vi "LSMcontroller_v64_updatedwaveformhandling.vi"() -> ()   [LabVIEW 2015] (continued)
                                tunnel: [_ w2837 _ w2843] -> w2785
                                frame 1 {
                                n478 = call "2pparameters.vi"("command"="get") -> ("params out"=w2797:T10)  [unwired: 1 in]
                                n479 = Unbundle By Name(w2797) -> ("wavdet"=w2798:bool, "sAOxy"=w2800:i32, "refwfsize"=w2801:dbl, "srate Img"=w2799:sgl)
                                n480 = call "waveformsDObuffer.vi"("command"="get") -> ("DO wf out"=w2793:digitalwaveform[])  [unwired: 1 in]
                                n481 = case shown="True" w2798 {
                                tunnel: [w2805 w2818] -> w2795
                                tunnel: w2799 -> [w2814 w2833]
                                tunnel: w2800 -> [w2804 w2824]
                                tunnel: w2801 -> [_ w2830]
                                frame False {
                                w2808 = u16 0 items=["unsigned binary", "offset binary", "2's complement"] ("data format (offset binary)")
                                n482 = Initialize Array(sgl 0.0, w2804) -> (w2811:sgl[])
                                n483 = Replace Array Subset(array=w2811, new element=sgl 1.0, index=0) -> (w2809:sgl[])
                                n484 = Reciprocal(x=w2814) -> (1/x=w2815:sgl)
                                n485 = Bundle By Name("Y"=w2809, "dt"=w2815) -> (w2806:waveform(sgl))  [unwired: 1 in]
                                n486 = call-poly <vilib>:"Analog to Digital.vi"("data format (offset binary)"=w2808, "compress digital (T)"=TRUE, "full-scale range (pk-pk)"=1.0, "resolution (16 bit)"=1, "analog waveform"=w2806) -> ("digital waveform"=w2805:digitalwaveform)  [unwired: 3 in, 3 out]
                                }
                                frame True {
                                w2821 = u16 0 items=["unsigned binary", "offset binary", "2's complement"] ("data format (offset binary)")
                                n487 = To Double Precision Float(number=w2824) -> (double precision float=w2831:dbl)
                                n488 = Initialize Array(sgl 0.0, w2824) -> (w2826:sgl[])
                                n489 = Divide(x=w2830, y=w2831) -> (x/y=w2828:dbl)
                                n490 = Round Toward +Infinity(x=w2828) -> (ceil(x): smallest int >= x=w2829:dbl)
                                n491 = Replace Array Subset(array=w2826, new element=sgl 1.0, index=0) -> (w2823:sgl[])
                                n492 = for {
                                N: w2829 -> [_]
                                tunnel: w2823 -> [w2835]
                                tunnel: [w2835] -> w2832 mode=concatenating
                                }
                                n493 = Reciprocal(x=w2833) -> (1/x=w2834:sgl)
                                n494 = Bundle By Name("Y"=w2832, "dt"=w2834) -> (w2819:waveform(sgl))  [unwired: 1 in]
                                n495 = call-poly <vilib>:"Analog to Digital.vi"("data format (offset binary)"=w2821, "compress digital (T)"=TRUE, "full-scale range (pk-pk)"=1.0, "resolution (16 bit)"=1, "analog waveform"=w2819) -> ("digital waveform"=w2818:digitalwaveform)  [unwired: 3 in, 3 out]
                                }
                                }
                                n496 = Build Array (concatenate)(w2793, w2795) -> (w2791:digitalwaveform[])
                                n497 = call "waveformsDObuffer.vi"("DO wf in"=w2791, "command"="set") -> ()  [unwired: 1 out]
                                }
                                frame 2 {
                                n498 = call "waveformsDObuffer.vi"("command"="get") -> ("DO wf out"=w2839:digitalwaveform[])  [unwired: 1 in]
                                n499 = Delete From Array(array=w2839, length=1, index=w2842) -> (deleted portion=w2837:digitalwaveform[], array with subset deleted=w2836:digitalwaveform[])
                                n500 = call "waveformsDObuffer.vi"("DO wf in"=w2836, "command"="set") -> ()  [unwired: 1 out]
                                }
                                frame 3, Default {
                                }
                                frame 0 {
                                n501 = local read "Measurement"() -> (w2845:T4)
                                n502 = To Unsigned Long Integer(number=w2845) -> (unsigned 32bit integer=w2844:u32)
                                n503 = case shown="5..7" w2844 {
                                tunnel: w2846 -> [_ w2849]
                                tunnel: [_ w2848] -> w2843
                                frame 0..4, Default {
                                }
                                frame 5..7 {
                                n504 = call "2pparameters.vi"("command"="get") -> ("params out"=w2856:T10)  [unwired: 1 in]
                                n505 = Unbundle By Name(w2856) -> ("wavdet"=w2857:bool, "sAOxy"=w2859:i32, "refwfsize"=w2860:dbl, "srate Img"=w2858:sgl)
                                n506 = call "waveformsDObuffer.vi"("command"="get") -> ("DO wf out"=w2850:digitalwaveform[])  [unwired: 1 in]
                                n507 = Index Array(array=w2850, index=w2849) -> (element=w2851:digitalwaveform)
                                n508 = case shown="True" w2857 {
                                tunnel: [w2864 w2877] -> w2854
                                tunnel: w2858 -> [w2873 w2892]
                                tunnel: w2859 -> [w2863 w2883]
                                tunnel: w2860 -> [_ w2889]
                                frame False {
                                w2867 = u16 0 items=["unsigned binary", "offset binary", "2's complement"] ("data format (offset binary)")
                                n509 = Initialize Array(sgl 0.0, w2863) -> (w2870:sgl[])
                                n510 = Replace Array Subset(array=w2870, new element=sgl 1.0, index=0) -> (w2868:sgl[])
                                n511 = Reciprocal(x=w2873) -> (1/x=w2874:sgl)
                                n512 = Bundle By Name("Y"=w2868, "dt"=w2874) -> (w2865:waveform(sgl))  [unwired: 1 in]
                                n513 = call-poly <vilib>:"Analog to Digital.vi"("data format (offset binary)"=w2867, "compress digital (T)"=TRUE, "full-scale range (pk-pk)"=1.0, "resolution (16 bit)"=1, "analog waveform"=w2865) -> ("digital waveform"=w2864:digitalwaveform)  [unwired: 3 in, 3 out]
                                }
                                frame True {
                                w2880 = u16 0 items=["unsigned binary", "offset binary", "2's complement"] ("data format (offset binary)")
                                n514 = To Double Precision Float(number=w2883) -> (double precision float=w2890:dbl)
                                n515 = Initialize Array(sgl 0.0, w2883) -> (w2885:sgl[])
                                n516 = Divide(x=w2889, y=w2890) -> (x/y=w2887:dbl)
                                n517 = Round Toward +Infinity(x=w2887) -> (ceil(x): smallest int >= x=w2888:dbl)
                                n518 = Replace Array Subset(array=w2885, new element=sgl 1.0, index=0) -> (w2882:sgl[])
                                n519 = for {
                                N: w2888 -> [_]
                                tunnel: w2882 -> [w2894]
                                tunnel: [w2894] -> w2891 mode=concatenating
                                }
                                n520 = Reciprocal(x=w2892) -> (1/x=w2893:sgl)
                                n521 = Bundle By Name("Y"=w2891, "dt"=w2893) -> (w2878:waveform(sgl))  [unwired: 1 in]
                                n522 = call-poly <vilib>:"Analog to Digital.vi"("data format (offset binary)"=w2880, "compress digital (T)"=TRUE, "full-scale range (pk-pk)"=1.0, "resolution (16 bit)"=1, "analog waveform"=w2878) -> ("digital waveform"=w2877:digitalwaveform)  [unwired: 3 in, 3 out]
                                }
                                }
                                n523 = Build Array(w2851) -> (w2848:digitalwaveform[])
                                n524 = Replace Array Subset(array=w2850, new element=w2854, index=w2849) -> (w2847:digitalwaveform[])
                                n525 = call "waveformsDObuffer.vi"("DO wf in"=w2847, "command"="set") -> ()  [unwired: 1 out]
                                }
                                }
                                }
                                }
                              }
                              frame #10 {
                                n526 = local read "Meastab"() -> (w2909:enum32{"X-Y Image", "Linescan", "Timetrace"})
                                n527 = property on="refwf" class="Ring (strict)"() -> ("RingText.Text"=w2906:string)  [unwired: 2 in, 2 out]
                                n528 = case shown="\"Timetrace\"" w2909 {
                                tunnel: [w2911 w2912] -> w2910
                                frame "X-Y Image", Default {
                                n529 = local read "Sampling rate"() -> (w2911:dbl)
                                }
                                frame "Timetrace" {
                                n530 = local read "srateAODOtt"() -> (w2912:dbl)
                                }
                                }
                                n531 = call "waveformsAObuffer.vi"("command"="get") -> ("AO wf out"=w2897:waveform(dbl)[])  [unwired: 1 in]
                                n532 = local read "wavdet"() -> (w2907:bool)
                                n533 = call "waveformsDObuffer.vi"("command"="get") -> ("DO wf out"=w2901:digitalwaveform[])  [unwired: 1 in]
                                n534 = call "correctwaveformsizetemp.vi"("new sampling frequency (Hz)"=w2910, "start"=TRUE, "reference waveforms to"=w2906, "Analog waveforms in"=w2897, "stop"=FALSE, "Digital waveforms in"=w2901) -> ("analog wf out"=w2903:waveform(dbl)[], "Digital wf out"=w2905:digitalwaveform[], "measpoints"=w2908:i32)
                                n535 = call "GetNumCamFramesv2.vi"("Digital Waveform Graph"=w2905) -> ("Numeric"=w2904:i32)  [unwired: 10 in]
                                n536 = call "waveformsDObuffer.vi"("DO wf in"=w2905, "command"="set") -> ()  [unwired: 1 out]
                                n537 = call "waveformsAObuffer.vi"("AO wf in"=w2903, "command"="set") -> ()  [unwired: 1 out]
                                n538 = local write "Total Camera Frames"(w2904) -> ()
                                n539 = case shown="True" w2907 {
                                tunnel: w2908 -> [_ w2913]
                                frame False {
                                }
                                frame True {
                                n540 = local write "# of frames"(w2913) -> ()
                                }
                                }
                              }
                            }
                          }
                          frame #6 {
                            # "Disabled for conversion to 64 bit"
                            n541 = disable-structure shown="Disabled" {
                              frame Disabled {
                                n542 = local read "Measurement"() -> (w2918:T4)
                                n543 = case shown="\"Lifetime (scan)\"" w2918 {
                                frame "X-Y-t movie", Default {
                                }
                                frame "Lifetime (scan)" {
                                # "total acquisition time"
                                n544 = call "2pparameters.vi"("command"="get") -> ("params out"=w2924:T10)  [unwired: 1 in]
                                n545 = Unbundle By Name(w2924) -> ("measpoints"=w2945:i32, "avpp"=w2946:i32, "sAOxy"=w2925:i32, "srate Img"=w2947:sgl)
                                n546 = Multiply(x=w2945, y=w2946) -> (x*y=w2943:i32)
                                n547 = To Double Precision Float(number=w2925) -> (double precision float=w2930:dbl)
                                n548 = Divide(x=w2930, y=w2947) -> (x/y=w2932:dbl)
                                n549 = To Double Precision Float(number=w2943) -> (double precision float=w2928:dbl)
                                n550 = local read "min phot"() -> (w2939:u32)
                                n551 = local read "expected c/s"() -> (w2940:dbl)
                                n552 = Multiply(x=w2928, y=w2932) -> (x*y=w2926:dbl)
                                n553 = Multiply(x=w2926, y=1000.0) -> (x*y=w2931:dbl)
                                n554 = local read "Ch1 ZeroX"() -> (w2937:i32)
                                n555 = local read "truncate"() -> (w2938:u32)
                                n556 = To Long Integer(number=w2931) -> (32bit integer=w2941:i32)
                                n557 = To Long Integer(number=w2940) -> (32bit integer=w2942:i32)
                                n558 = local read "Number of Bins"() -> (w2933:u32)
                                n559 = local read "Ch1 Level"() -> (w2935:i32)
                                n560 = local read "Ch0 ZeroX"() -> (w2936:i32)
                                n561 = local write "Acquisition time"(w2941) -> ()
                                n562 = local read "Ch0 Level"() -> (w2934:i32)
                                n563 = call "lifetimeparameters.vi"("command"="get") -> ("Params out"=w2922:T19)  [unwired: 1 in]
                                n564 = Add(x=10, y=w2941) -> (x+y=w2929:i32)
                                n565 = Bundle By Name(cluster=w2922, "acq time"=w2929, "acq rate"=w2942, "# bins"=w2933, "Ch0 Level"=w2934, "Ch1 Level"=w2935, "Ch0 ZeroX"=w2936, "Ch1 ZeroX"=w2937, "min photons"=w2939, "truncate"=w2938) -> (w2921:T19)
                                n566 = local write "Acquisition rate"(w2942) -> ()
                                n567 = call "lifetimeparameters.vi"("Params in"=w2921, "command"="set") -> ()  [unwired: 1 out]
                                }
                                }
                                n568 = local read "min phot"() -> (w2916:u32)
                                n569 = Decrement(x=w2916) -> (x-1=w2917:u32)
                                n570 = To Double Precision Float(number=w2917) -> (double precision float=w2915:dbl)
                                n571 = property on="img_CH1" class="IntGraph (strict)"("ZScale.Minimum"=w2915) -> ()  [unwired: 2 in, 2 out]
                              }
                              frame Enabled {
                              }
                            }
                            n572 = local write "64bit disabled"(TRUE ("64bit disabled")) -> ()
                          }
                          frame #7 {
                            n573 = local read "Sampling rate"() -> (w2949:dbl)
                            n574 = call "calcdaqtime.vi"("sampling rate"=w2949) -> ("Calc. time per frame (ms)"=w2948:dbl)
                            n575 = local write "Calc. time per frame (ms)"(w2948) -> ()
                          }
                          frame #8 {
                            n576 = call "2pparameters.vi"("command"="get") -> ("params out"=w2960:T10)  [unwired: 1 in]
                            n577 = local read "Measurement"() -> (w2951:T4)
                            n578 = Unbundle By Name(w2960) -> ("bufferAI"=w2958:i32, "srate"=w2959:sgl)
                            n579 = To Double Precision Float(number=w2958) -> (double precision float=w2952:dbl)
                            n580 = To Double Precision Float(number=w2959) -> (double precision float=w2962:dbl)
                            n581 = case shown="\"X-Y-t movie\", Default" w2951 {
                              tunnel: [w2967 w2971] -> w2950
                              frame "X-Y-t movie", Default {
                                n582 = local read "wavdet"() -> (w2968:bool)
                                n583 = case shown="False" w2968 {
                                tunnel: [w2969 w2970] -> w2967
                                frame False {
                                w2969 = 10123 items=["Finite Samples"=10178, "Continuous Samples"=10123, "Hardware Timed Single Point"=12522] ("sample mode")
                                }
                                frame True {
                                w2970 = 10123 items=["Finite Samples"=10178, "Continuous Samples"=10123, "Hardware Timed Single Point"=12522] ("sample mode")
                                }
                                }
                              }
                              frame "X-Y-Z stack" {
                                w2971 = 10178 items=["Finite Samples"=10178, "Continuous Samples"=10123, "Hardware Timed Single Point"=12522] ("sample mode")
                              }
                            }
                            n584 = Divide(x=w2952, y=w2962) -> (x/y=w2966:dbl)
                            n585 = Multiply(x=w2966, y=2.0) -> (x*y=w2963:dbl)
                            n586 = Max & Min(x=w2963, y=10.0) -> (max(x,y)=w2953:dbl)  [unwired: 1 out]
                            n587 = call "2pparameters.vi"("command"="get") -> ("params out"=w2957:T10)  [unwired: 1 in]
                            n588 = Bundle By Name(cluster=w2957, "timeout"=w2953, "sample mode"=w2950) -> (w2954:T10)
                            n589 = call "2pparameters.vi"("Params in"=w2954, "command"="set") -> ()  [unwired: 1 out]
                          }
                          frame #9 {
                            n590 = local read "# of frames"() -> (w2972:i32)
                            n591 = call "timestamps.vi"("# of frames"=w2972, "command"="init") -> ()  [unwired: 2 in, 1 out]
                          }
                        }
                      }
                      frame #2 {
                        # "Disabled for conversion to 64 bit"
                        n592 = call "prepAO_img.vi"() -> ("Terminal Name with Device Prefix"=w2975:tag)
                        n593 = call "prepAI_img.vi"("triggersource"=w2975) -> ()  [unwired: 2 in]
                        n594 = call "prepCI_img.vi"("ArmStart.DigEdge.Src"=w2975) -> ()  [unwired: 1 in]
                        n595 = call "prepDO_img.vi"() -> ()  [unwired: 2 in]
                        n596 = disable-structure shown="Disabled" {
                          frame Disabled {
                            n597 = local read "Measurement"() -> (w2976:T4)
                            n598 = case shown="\"Lifetime (scan)\"" w2976 {
                              frame "X-Y-t movie", Default {
                              }
                              frame "Lifetime (scan)" {
                                n599 = stacked-sequence {
                                frame #0 {
                                n600 = call "PH-temp.vi"("String"="clear" ("command")) -> ()  [unwired: 2 in, 2 out]
                                n601 = call "PH-temp-raw.vi"("command"="empty") -> ()  [unwired: 1 in, 1 out]
                                }
                                frame #1 {
                                n602 = call "calib.vi"() -> ()  [unwired: 1 in]
                                }
                                frame #2 {
                                n603 = call "setup.vi"() -> ()  [unwired: 1 in]
                                }
                                }
                              }
                            }
                          }
                          frame Enabled {
                          }
                        }
                        n604 = local write "64bit disabled"(TRUE ("64bit disabled")) -> ()
                      }
                      frame #3 {
                        n605 = local read "save\ndata"() -> (w2979:bool)
                        n606 = case shown="True" w2979 {
                          tunnel: w2980 -> [_ w2984]
                          frame False {
                          }
                          frame True {
                            n607 = local read "filename prefix"() -> (w2982:string)
                            n608 = local read "data dir"() -> (w2983:path)
                            n609 = call "preparetiffs.vi"("filename prefix"=w2982, "data dir"=w2983, "timestamp"=w2984) -> ("full-filename"=w2981:string)  [unwired: 1 in]
                            n610 = local write "full-filename"(w2981) -> ()
                          }
                        }
                        n611 = call "preptempbuffers.vi"() -> ()  [unwired: 12 in]
                      }
                      frame #4 {
                        # "Disabled Thorlabs Zstage;\nneeds to be replaced by PI code"
                        n612 = local read "Measurement"() -> (w2985:T4)
                        n613 = case shown="\"X-Y-Z stack\"" w2985 {
                          frame "X-Y-t movie", Default {
                          }
                          frame "X-Y-Z stack" {
                            # "Move Z stage"
                            n614 = stacked-sequence {
                              seq-local: [w2987 _] -> [_ w3000]
                              frame #0 {
                                n615 = local read "Z-Start (um)"() -> (w2991:dbl)
                                n616 = local read "Z-end (um)"() -> (w2990:dbl)
                                n617 = local read "# of frames"() -> (w2992:i32)
                                n618 = call "calcZslice.vi"("current slice"=0, "# of Slices"=w2992, "Z-Start (um)"=w2991, "Z-end (um)"=w2990) -> ("zpos (V)"=w2988:dbl, "zpos (um)"=w2987:dbl)
                                n619 = call "moveZ_V2.vi"("Z"=w2988) -> ()
                                n620 = local write "Cal. Z"(w2987) -> ()
                              }
                              frame #1 {
                                n621 = local read "Pstart"() -> (w2999:dbl)
                                n622 = local read "Pend"() -> (w2998:dbl)
                                n623 = local read "exp?"() -> (w2997:bool)
                                n624 = local read "Z-Start (um)"() -> (w3002:dbl)
                                n625 = local read "Z0"() -> (w3003:dbl)
                                n626 = local read "Z-end (um)"() -> (w3001:dbl)
                                n627 = local read "wavelength(nm)"() -> (w2996:dbl)
                                n628 = local read "# of frames"() -> (w2995:i32)
                                n629 = call "pockelscellzstage.vi"("current slice"=0, "# of Slices"=w2995, "wavelength (nm)"=w2996, "Z0"=w3003, "exp?"=w2997, "Zstart"=w3002, "Pend"=w2998, "Pstart"=w2999, "Z"=w3000, "Zend"=w3001) -> ("T(%)"=w2993:dbl)  [unwired: 1 in]
                                n630 = property on="Laserpower \n(%)" class="Slide (strict)"("Value"=w2993) -> ()  [unwired: 2 in, 2 out]
                                n631 = property on="lpow" class="DigNum (strict)"("Value"=w2993) -> ()  [unwired: 2 in, 2 out]
                              }
                            }
                          }
                        }
                        n632 = local write "Thorlabs Zstage disabled"(TRUE ("64bit disabled")) -> ()
                      }
                      frame #5 {
                        n633 = flat-sequence {
                          frame #0 {
                            n634 = call "2pparameters.vi"("command"="get") -> ("params out"=w3005:T10)  [unwired: 1 in]
                            n635 = Unbundle By Name(w3005) -> ("autoshutter"=w3006:bool)
                            n636 = case shown="True" w3006 {
                              frame False {
                              }
                              frame True {
                                n637 = call "shuttercontrol.vi"("command"="open") -> ()  [unwired: 1 in, 1 out]
                              }
                            }
                          }
                          frame #1 {
                            n638 = call "2pparameters.vi"("command"="get") -> ("params out"=w3010:T10)  [unwired: 1 in]
                            n639 = Tick Count (ms)() -> (millisecond timer value=w3009:u32)
                            n640 = Bundle By Name(cluster=w3010, "starttick"=w3009) -> (w3008:T10)
                            n641 = call "2pparameters.vi"("Params in"=w3008, "command"="set") -> ()  [unwired: 1 out]
                          }
                        }
                      }
                      frame #6 {
                        n642 = local read "Measurement"() -> (w3013:T4)
                        n643 = case shown="\"Lifetime (scan)\"" w3013 {
                          frame "X-Y-t movie" {
                            n644 = flat-sequence {
                              frame #0 {
                                n645 = call "runAI_img.vi"() -> ()  [unwired: 12 in]
                                n646 = call "runCI.vi"() -> ()  [unwired: 12 in]
                                n647 = call "runDO_img.vi"() -> ()  [unwired: 12 in]
                              }
                              frame #1 {
                                n648 = call "runAO_img.vi"() -> ()  [unwired: 12 in]
                              }
                            }
                          }
                          frame "Lifetime (scan)" {
                            # "Disabled for conversion to 64 bit"
                            n649 = disable-structure shown="Disabled" {
                              frame Disabled {
                                n650 = flat-sequence {
                                frame #0 {
                                n651 = call "runLT_img.vi"() -> ()  [unwired: 1 in]
                                n652 = call "runDO_img.vi"() -> ()  [unwired: 12 in]
                                }
                                frame #1 {
                                n653 = call "runAI_img.vi"() -> ()  [unwired: 12 in]
                                n654 = call "runCI.vi"() -> ()  [unwired: 12 in]
                                }
                                frame #2 {
                                n655 = call "runAO_img.vi"() -> ()  [unwired: 12 in]
                                }
                                }
                              }
                              frame Enabled {
                              }
                            }
                            n656 = local write "64bit disabled"(TRUE ("64bit disabled")) -> ()
                          }
                          frame "X-Y-Z stack", Default {
                          }
                        }
                      }
                      frame #7 {
                        # "Disabled for conversion to 64 bit"
                        n657 = while {
                          i -> [w3042]
                          stop <- w3039 stop-if-true
                          n658 = local read "Exit"() -> (w3047:bool)
                          n659 = local read "Stop"() -> (w3038:bool)
                          n660 = Or(x=w3038, y=w3047) -> (x .or. y?=w3043:bool)
                          n661 = case shown="False" w3043 {
                            tunnel: w3042 -> [w3048 _]
                            frame False {
                              n662 = stacked-sequence {
                                seq-local: [w3050 _ _ _ _ _ _] -> [_ _ _ _ _ _ w3179]
                                seq-local: [w3049 _ _ _ _ _ _] -> [_ _ _ _ _ _ w3178]
                                tunnel: w3048 -> [_ w3056 _ _ _ _ _]
                                frame #0 {
                                n663 = local read "Live"() -> (w3051:bool)
                                n664 = case shown="True" w3051 {
                                tunnel: [_ w3053] -> w3050
                                tunnel: [_ w3052] -> w3049
                                frame False {
                                }
                                frame True {
                                n665 = local read "Laserpower \n(%)"() -> (w3052:dbl)
                                n666 = local read "lpow"() -> (w3053:dbl)
                                }
                                }
                                n667 = call "preptempbuffers.vi"() -> ()  [unwired: 12 in]
                                }
                                frame #1 {
                                # "Move in Z if necessary"
                                # "Disabled Thorlabs Zstage;\nneeds to be replaced by PI code"
                                n668 = local read "Measurement"() -> (w3054:T4)
                                n669 = case shown="\"X-Y-Z stack\"" w3054 {
                                tunnel: w3056 -> [_ w3057]
                                frame "X-Y-t movie", Default {
                                }
                                frame "X-Y-Z stack" {
                                n670 = stacked-sequence {
                                seq-local: [w3058 _] -> [_ w3066]
                                tunnel: w3057 -> [w3060 w3065]
                                frame #0 {
                                n671 = local read "Z-Start (um)"() -> (w3062:dbl)
                                n672 = local read "Z-end (um)"() -> (w3061:dbl)
                                n673 = local read "# of frames"() -> (w3063:i32)
                                n674 = call "calcZslice.vi"("current slice"=w3060, "# of Slices"=w3063, "Z-Start (um)"=w3062, "Z-end (um)"=w3061) -> ("zpos (V)"=w3059:dbl, "zpos (um)"=w3058:dbl)
                                n675 = local write "Cal. Z"(w3058) -> ()
                                n676 = call "moveZ_V2.vi"("Z"=w3059) -> ()
                                }
                                frame #1 {
                                n677 = local read "Pstart"() -> (w3071:dbl)
                                n678 = local read "Pend"() -> (w3070:dbl)
                                n679 = local read "exp?"() -> (w3069:bool)
                                n680 = local read "Z-Start (um)"() -> (w3073:dbl)
                                n681 = local read "Z0"() -> (w3074:dbl)
                                n682 = local read "Z-end (um)"() -> (w3072:dbl)
                                n683 = local read "wavelength(nm)"() -> (w3068:dbl)
                                n684 = local read "# of frames"() -> (w3067:i32)
                                n685 = call "pockelscellzstage.vi"("current slice"=w3065, "# of Slices"=w3067, "wavelength (nm)"=w3068, "Z0"=w3074, "exp?"=w3069, "Zstart"=w3073, "Pend"=w3070, "Pstart"=w3071, "Z"=w3066, "Zend"=w3072) -> ("T(%)"=w3064:dbl)  [unwired: 1 in]
                                n686 = property on="Laserpower \n(%)" class="Slide (strict)"("Value"=w3064) -> ()  [unwired: 2 in, 2 out]
                                n687 = property on="lpow" class="DigNum (strict)"("Value"=w3064) -> ()  [unwired: 2 in, 2 out]
                                }
                                }
                                }
                                }
                                n688 = local write "Thorlabs Zstage disabled"(TRUE ("64bit disabled")) -> ()
                                }
                                frame #2 {
                                # "main loop"
                                n689 = for {
                                N: "avpp" -> [_]
                                i -> [w3080]
                                n690 = local read "Stop"() -> (w3078:bool)
                                n691 = local read "Exit"() -> (w3077:bool)
                                n692 = Increment(x=w3080) -> (x+1=w3079:i32)
                                n693 = Or(x=w3078, y=w3077) -> (x .or. y?=w3076:bool)
                                n694 = case shown="False" w3076 {
                                tunnel: w3079 -> [w3081 _]
                                frame False {
                                n695 = stacked-sequence {
                                seq-local: [w3082 _ _ _ _ _ _] -> [_ _ _ w3095 w3107 w3115 _]
                                tunnel: w3081 -> [w3083 _ _ _ _ _ _]
                                frame #0 {
                                n696 = local read "Live"() -> (w3082:bool)
                                n697 = case shown="True" w3082 {
                                tunnel: w3083 -> [_ w3086]
                                frame False {
                                }
                                frame True {
                                # "collect timetag for current image\nplus curent average"
                                n698 = To Single Precision Float(number=w3086) -> (single precision float=w3084:sgl)
                                n699 = Tick Count (ms)() -> (millisecond timer value=w3085:u32)
                                n700 = local write "Tick for Frame"(w3085) -> ()
                                n701 = local write "Current Average"(w3084) -> ()
                                }
                                }
                                }
                                frame #1 {
                                n702 = local read "Measurement"() -> (w3087:T4)
                                n703 = case shown="\"X-Y-Z stack\"" w3087 {
                                frame "X-Y-t movie", Default {
                                }
                                frame "X-Y-Z stack" {
                                n704 = stacked-sequence {
                                frame #0 {
                                n705 = disable-structure shown="Disabled" {
                                frame Disabled {
                                n706 = call "2pparameters.vi"("command"="get") -> ("params out"=w3089:T10)  [unwired: 1 in]
                                n707 = Unbundle By Name(w3089) -> ("autoshutter"=w3090:bool)
                                n708 = case shown="True" w3090 {
                                frame False {
                                }
                                frame True {
                                n709 = call "shuttercontrol.vi"("command"="open") -> ()  [unwired: 1 in, 1 out]
                                }
                                }
                                }
                                frame Enabled {
                                }
                                }
                                }
                                frame #1 {
                                n710 = call "runAI_img.vi"() -> ()  [unwired: 12 in]
                                n711 = call "runCI.vi"() -> ()  [unwired: 12 in]
                                n712 = call "runDO_img.vi"() -> ()  [unwired: 12 in]
                                }
                                frame #2 {
                                n713 = call "runAO_img.vi"() -> ()  [unwired: 12 in]
                                }
                                }
                                }
                                }
                                }
                                frame #2 {
                                n714 = call "collectCI_img.vi"() -> ("Avg cts/s"=w3094:dbl, "recorded samples"=w3093:i32)  [unwired: 1 out]
                                n715 = call "collectAI_img.vi"() -> ("wrap"=w3092:i32)  [unwired: 3 in]
                                n716 = local write "scol"(w3093) -> ()
                                n717 = local write "wrap"(w3092) -> ()
                                n718 = local write "Avg Counts/s"(w3094) -> ()
                                }
                                frame #3 {
                                n719 = case shown="True" w3095 {
                                frame False {
                                }
                                frame True {
                                n720 = local read "Measurement"() -> (w3096:T4)
                                n721 = case shown="\"X-Y-t movie\", Default" w3096 {
                                frame "X-Y-t movie", Default {
                                n722 = local read "ROI Type"() -> (w3097:u16)
                                n723 = case shown="0" w3097 {
                                frame 0 {
                                # "display chosen channels"
                                n724 = local read "Current Average"() -> (w3106:sgl)
                                n725 = local read "image1list"() -> (w3102:u16)
                                n726 = local read "image2list"() -> (w3105:u16)
                                n727 = To Unsigned Word Integer(number=w3105) -> (unsigned 16bit integer=w3100:u16)
                                n728 = To Unsigned Word Integer(number=w3102) -> (unsigned 16bit integer=w3101:u16)
                                n729 = call "dattoimage.vi"("image2list"=w3100, "Current Average"=w3106, "image1list"=w3101) -> ("image 2 array out"=w3104:sgl[][], "image 1 array out"=w3103:sgl[][])
                                n730 = Transpose 2D Array(2D array=w3103) -> (transposed array=w3099:sgl[][])
                                n731 = Transpose 2D Array(2D array=w3104) -> (transposed array=w3098:sgl[][])
                                n732 = local write "img_CH1"(w3099) -> ()
                                n733 = local write "img_CH2"(w3098) -> ()
                                }
                                frame 1, Default {
                                }
                                }
                                }
                                frame "Lifetime (scan)" {
                                }
                                }
                                }
                                }
                                }
                                frame #4 {
                                n734 = case shown="True" w3107 {
                                frame False {
                                }
                                frame True {
                                # "set colormaps"
                                n735 = call "misc-global.vi"("command"="get") -> ("misc out"=w3111:cluster{"Colormaps":u32[][]})  [unwired: 1 in]
                                n736 = Unbundle By Name(w3111) -> ("Colormaps"=w3110:u32[][])
                                n737 = control-ref of="img_CH1"() -> (w3114:refnum<vi>)
                                n738 = control-ref of="img_CH2"() -> (w3113:refnum<vi>)
                                n739 = Index Array(array=w3110, index (row)="Colormap") -> (element=w3109:u32[])  [unwired: 1 in]
                                n740 = property class="IntGraph (strict)"(reference=w3114, "Color Table"=w3109) -> ()  [unwired: 1 in, 2 out]
                                n741 = property class="IntGraph (strict)"(reference=w3113, "Color Table"=w3109) -> ()  [unwired: 1 in, 2 out]
                                }
                                }
                                }
                                frame #5 {
                                n742 = case shown="True" w3115 {
                                frame False {
                                }
                                frame True {
                                # "crude estimate of time per frame\n(resolution is 1 ms), not so much for\nplotting purposes, more for debugging\ncollection and processing data"
                                n743 = local read "ypixels ref"() -> (w3120:i32)
                                n744 = local read "Tick for Frame"() -> (w3121:u32)
                                n745 = Tick Count (ms)() -> (millisecond timer value=w3122:u32)
                                n746 = To Double Precision Float(number=w3120) -> (double precision float=w3119:dbl)
                                n747 = Subtract(x=w3122, y=w3121) -> (x-y=w3117:u32)
                                n748 = To Double Precision Float(number=w3117) -> (double precision float=w3118:dbl)
                                n749 = local write "Meas. time per frame (ms)"(w3117) -> ()
                                n750 = Divide(x=w3118, y=w3119) -> (x/y=w3116:dbl)
                                n751 = local write "time per line (ms)"(w3116) -> ()
                                }
                                }
                                }
                                frame #6 {
                                n752 = local read "Measurement"() -> (w3123:T4)
                                n753 = case shown="\"X-Y-Z stack\"" w3123 {
                                frame "X-Y-t movie", Default {
                                }
                                frame "X-Y-Z stack" {
                                n754 = call "2pparameters.vi"("command"="get") -> ("params out"=w3125:T10)  [unwired: 1 in]
                                n755 = Unbundle By Name(w3125) -> ("autoshutter"=w3126:bool)
                                n756 = call "stopCI_img.vi"() -> ()  [unwired: 12 in]
                                n757 = call "stopAI_img.vi"() -> ()  [unwired: 12 in]
                                n758 = case shown="True" w3126 {
                                frame False {
                                }
                                frame True {
                                n759 = call "shuttercontrol.vi"("command"="close") -> ()  [unwired: 1 in, 1 out]
                                }
                                }
                                n760 = Wait (ms)(milliseconds to wait=u32 100) -> ()  [unwired: 1 out]
                                n761 = call "stopAO_img.vi"() -> ()  [unwired: 12 in]
                                n762 = call "stopDO_img.vi"() -> ()  [unwired: 12 in]
                                }
                                }
                                }
                                }
                                }
                                frame True {
                                }
                                }
                                }
                                }
                                frame #3 {
                                n763 = local read "Measurement"() -> (w3129:T4)
                                n764 = case shown="\"Lifetime (scan)\"" w3129 {
                                frame "X-Y-t movie", Default {
                                }
                                frame "Lifetime (scan)" {
                                w3132 = u16 2 items=["Stream to disk", "Post process", "real time process"] ("Ring")
                                n765 = local read "T3R Data processing"() -> (w3133:u16)
                                n766 = Equal?(x=w3133, y=w3132) -> (x = y?=w3131:bool)
                                n767 = case shown="True" w3131 {
                                frame False {
                                }
                                frame True {
                                n768 = disable-structure shown="Disabled" {
                                frame Disabled {
                                n769 = local read "lineshift"() -> (w3136:i32)
                                n770 = call "wrapcutlifetime.vi"("lineshift"=w3136) -> ("pt3img"=w3138:u16[][], "lifetimes"=w3137:sgl[][], "okay"=w3134:bool, "# of frames"=w3135:i32)
                                n771 = case shown="True" w3134 {
                                tunnel: w3138 -> [_ w3148]
                                tunnel: w3137 -> [_ w3146]
                                tunnel: w3135 -> [_ w3142]
                                frame False {
                                }
                                frame True {
                                # "lifetime"
                                # "intensity"
                                n772 = Transpose 2D Array(2D array=w3148) -> (transposed array=w3140:u16[][])
                                n773 = Transpose 2D Array(2D array=w3146) -> (transposed array=w3147:sgl[][])
                                n774 = local write "frames recorded"(w3142) -> ()
                                n775 = local read "counts"() -> (w3141:i32)
                                n776 = Array Max & Min(array=w3140) -> (max value=w3145:u16)  [unwired: 3 out]
                                n777 = To Single Precision Float(number=w3140) -> (single precision float=w3139:sgl[][])
                                n778 = local write "img_CH2"(w3147) -> ()
                                n779 = local write "img_CH1"(w3139) -> ()
                                n780 = Quotient & Remainder(x=w3141, y=w3142) -> (floor(x/y)=→"photons/frame":i32)  [unwired: 1 out]
                                n781 = To Double Precision Float(number=w3145) -> (double precision float=w3144:dbl)
                                n782 = property on="img_CH1" class="IntGraph (strict)"("ZScale.Maximum"=w3144) -> ()  [unwired: 2 in, 2 out]
                                }
                                }
                                }
                                frame Enabled {
                                }
                                }
                                }
                                }
                                }
                                }
                                n783 = local read "save\ndata"() -> (w3130:bool)
                                n784 = case shown="True" w3130 {
                                frame False {
                                }
                                frame True {
                                n785 = local read "Current Average"() -> (w3149:sgl)
                                n786 = call "savetiffs.vi"("current average"=w3149) -> ()
                                }
                                }
                                }
                                frame #4 {
                                n787 = local read "save\ndata"() -> (w3150:bool)
                                n788 = case shown="True" w3150 {
                                frame False {
                                }
                                frame True {
                                n789 = local read "points recorded"() -> (w3152:i32)
                                n790 = call "timestamps.vi"("points recorded"=w3152, "command"="add") -> ()  [unwired: 2 in, 1 out]
                                }
                                }
                                }
                                frame #5 {
                                n791 = local read "Live"() -> (w3153:bool)
                                n792 = case shown="True" w3153 {
                                frame False {
                                }
                                frame True {
                                n793 = local read "downright"() -> (w3158:bool)
                                n794 = local read "downleft"() -> (w3160:bool)
                                n795 = local read "upright"() -> (w3156:bool)
                                n796 = local read "upleft"() -> (w3154:bool)
                                n797 = local read "down"() -> (w3159:bool)
                                n798 = local read "right"() -> (w3157:bool)
                                n799 = local read "left"() -> (w3161:bool)
                                n800 = local read "up"() -> (w3155:bool)
                                n801 = Compound Arithmetic op=OR(w3154, w3155, w3156, w3157, w3158, w3159, w3160, w3161) -> (w3162:bool)
                                n802 = case shown="True" w3162 {
                                frame False {
                                }
                                frame True {
                                n803 = stacked-sequence {
                                frame #0 {
                                n804 = local read "downright"() -> (w3164:bool)
                                n805 = local read "downleft"() -> (w3166:bool)
                                n806 = local read "BigSmall"() -> (w3163:bool)
                                n807 = local read "upright"() -> (w3168:bool)
                                n808 = local read "upleft"() -> (w3171:bool)
                                n809 = local read "down"() -> (w3167:bool)
                                n810 = local read "right"() -> (w3169:bool)
                                n811 = local read "left"() -> (w3165:bool)
                                n812 = local read "up"() -> (w3170:bool)
                                n813 = call "movestageparams.vi"("command"="get") -> ("Params out"=w3174:T20)  [unwired: 1 in]
                                n814 = Bundle By Name(cluster=w3174, "upleft"=w3171, "up"=w3170, "upright"=w3168, "right"=w3169, "downright"=w3164, "down"=w3167, "downleft"=w3166, "left"=w3165, "Bigsmall"=w3163) -> (w3175:T20)
                                n815 = call "movestageparams.vi"("Params in"=w3175, "command"="set") -> ()  [unwired: 1 out]
                                }
                                frame #1 {
                                n816 = call "movestage.vi"() -> ()  [unwired: 12 in]
                                }
                                frame #2 {
                                w3176 = FALSE ("OK Button")
                                w3177 = FALSE ("OK Button")
                                n817 = property on="down" class="Bool (strict)"("Value"=w3177) -> ()  [unwired: 2 in, 2 out]
                                n818 = property on="up" class="Bool (strict)"("Value"=w3177) -> ()  [unwired: 2 in, 2 out]
                                n819 = property on="right" class="Bool (strict)"("Value"=w3177) -> ()  [unwired: 2 in, 2 out]
                                n820 = property on="left" class="Bool (strict)"("Value"=w3177) -> ()  [unwired: 2 in, 2 out]
                                n821 = property on="upright" class="Bool (strict)"("Value"=w3176) -> ()  [unwired: 2 in, 2 out]
                                n822 = property on="downleft" class="Bool (strict)"("Value"=w3176) -> ()  [unwired: 2 in, 2 out]
                                n823 = property on="downright" class="Bool (strict)"("Value"=w3176) -> ()  [unwired: 2 in, 2 out]
                                n824 = property on="upleft" class="Bool (strict)"("Value"=w3176) -> ()  [unwired: 2 in, 2 out]
                                }
                                }
                                }
                                }
                                }
                                }
                                }
                                frame #6 {
                                n825 = local read "Live"() -> (w3180:bool)
                                n826 = case shown="True" w3180 {
                                tunnel: w3179 -> [_ w3187]
                                tunnel: w3178 -> [_ w3186]
                                frame False {
                                }
                                frame True {
                                n827 = local read "Laserpower \n(%)"() -> (w3182:dbl)
                                n828 = local read "lpow"() -> (w3181:dbl)
                                n829 = Not Equal?(x=w3181, y=w3187) -> (x != y?=w3183:bool)
                                n830 = Not Equal?(x=w3182, y=w3186) -> (x != y?=w3184:bool)
                                n831 = Or(x=w3184, y=w3183) -> (x .or. y?=w3185:bool)
                                n832 = case shown="True" w3185 {
                                tunnel: w3184 -> [_ w3191]
                                tunnel: w3183 -> [_ w3190]
                                tunnel: w3182 -> [_ w3189]
                                tunnel: w3181 -> [_ w3188]
                                frame False {
                                }
                                frame True {
                                n833 = case shown="True" w3191 {
                                tunnel: w3189 -> [_ w3194]
                                frame False {
                                }
                                frame True {
                                n834 = local read "wavelength(nm)"() -> (w3195:dbl)
                                n835 = call "setpockelscellT.vi"("wavelength(nm)"=w3195, "transmission"=w3194) -> ()  [unwired: 1 in]
                                n836 = property on="lpow" class="DigNum (strict)"("Value"=w3194) -> ()  [unwired: 2 in, 2 out]
                                }
                                }
                                n837 = case shown="True" w3190 {
                                tunnel: w3188 -> [_ w3192]
                                frame False {
                                }
                                frame True {
                                n838 = local read "wavelength(nm)"() -> (w3193:dbl)
                                n839 = call "setpockelscellT.vi"("wavelength(nm)"=w3193, "transmission"=w3192) -> ()  [unwired: 1 in]
                                n840 = property on="Laserpower \n(%)" class="Slide (strict)"("Value"=w3192) -> ()  [unwired: 2 in, 2 out]
                                }
                                }
                                }
                                }
                                }
                                }
                                }
                              }
                            }
                            frame True {
                            }
                          }
                          n841 = Increment(x=w3042) -> (x+1=w3041:i32)
                          "points recorded" <- w3041
                          n842 = call "stopcond.vi"("prec"=w3041) -> ("stop"=w3040:bool)
                          n843 = local read "Stop"() -> (w3046:bool)
                          n844 = local read "Exit"() -> (w3045:bool)
                          n845 = Or(x=w3046, y=w3045) -> (x .or. y?=w3044:bool)
                          n846 = Or(x=w3040, y=w3044) -> (x .or. y?=w3039:bool)
                        }
                        n847 = disable-structure shown="Disabled" {
                          disable-tunnel: w3016 -> [w3022 _]
                          frame Disabled {
                            w3019 = u16 0 items=["Stream to disk", "Post process", "real time process"] ("Ring")
                            n848 = local read "T3R Data processing"() -> (w3018:u16)
                            n849 = Equal?(x=w3018, y=w3019) -> (x = y?=w3017:bool)
                            n850 = local read "save\ndata"() -> (w3021:bool)
                            n851 = local read "Measurement"() -> (w3023:T4)
                            n852 = And(x=w3021, y=w3017) -> (x .and. y?=w3020:bool)
                            n853 = case shown="\"Lifetime (scan)\"" w3023 {
                              tunnel: w3022 -> [_ w3027]
                              tunnel: w3020 -> [_ w3026]
                              frame "X-Y-t movie", Default {
                              }
                              frame "Lifetime (scan)" {
                                n854 = case shown="True" w3026 {
                                selector: w3026 -> [w3028 w3033]
                                tunnel: w3027 -> [_ w3031]
                                tunnel: [path "" ("appended path") w3034] -> w3025
                                tunnel: [w3028 w3033] -> w3024
                                frame False {
                                }
                                frame True {
                                n855 = local read "filename prefix"() -> (w3032:string)
                                n856 = local read "data dir"() -> (w3035:path)
                                n857 = call "generatedatafilename.vi"("timestamp"=w3031, "filename prefix in"=w3032) -> ("full-filename"=w3030:string)
                                n858 = Concatenate Strings(w3030, ".lvpt3img" ("string")) -> (w3037:string)
                                n859 = Build Path(base path=w3035, name or relative path=w3037) -> (appended path=w3034:path)
                                }
                                }
                                n860 = call "collectLT_img_v2.vi"("stream?"=w3024, "data file"=w3025) -> ()  [unwired: 2 out]
                              }
                            }
                          }
                          frame Enabled {
                          }
                        }
                        n861 = local write "64bit disabled"(TRUE ("64bit disabled")) -> ()
                      }
                      frame #8 {
                        # "Disabled for conversion to 64 bit"
                        n862 = local read "Measurement"() -> (w3198:T4)
                        n863 = case shown="\"Lifetime (scan)\"" w3198 {
                          tunnel: w3197 -> [_ _ w3199]
                          frame "X-Y-t movie", Default {
                          }
                          frame "X-Y-Z stack" {
                            n864 = call "eraseDO_img.vi"() -> ()  [unwired: 12 in]
                            n865 = call "eraseAO_img.vi"() -> ()  [unwired: 12 in]
                            n866 = call "eraseCI_img.vi"() -> ()  [unwired: 12 in]
                            n867 = call "eraseAI_img.vi"() -> ()  [unwired: 12 in]
                          }
                          frame "Lifetime (scan)" {
                            n868 = disable-structure shown="Disabled" {
                              disable-tunnel: w3199 -> [w3200 _]
                              frame Disabled {
                                n869 = stacked-sequence {
                                tunnel: w3200 -> [_ _ w3214 _ _]
                                frame #0 {
                                n870 = disable-structure shown="Disabled" {
                                frame Disabled {
                                n871 = call "stoperaseCI.vi"() -> ()  [unwired: 12 in]
                                n872 = call "stoperaseDO_img.vi"() -> ()  [unwired: 12 in]
                                n873 = call "stoperaseAO_img.vi"() -> ()  [unwired: 12 in]
                                n874 = call "stoperaseAI_img.vi"() -> ()  [unwired: 12 in]
                                }
                                frame Enabled {
                                }
                                }
                                }
                                frame #1 {
                                n875 = disable-structure shown="Disabled" {
                                frame Disabled {
                                n876 = local read "Acquisition time"() -> (w3204:i32)
                                n877 = call "collect_allLT_img.vi"() -> ("counts"=w3206:i32)  [unwired: 1 out]
                                n878 = local read "counts"() -> (w3207:i32)
                                n879 = Add(x=w3207, y=w3206) -> (x+y=w3205:i32)
                                "counts" <- w3205
                                n880 = Divide(x=w3205, y=w3204) -> (x/y=w3203:dbl)
                                n881 = Multiply(x=1000.0, y=w3203) -> (x*y=w3202:dbl)
                                n882 = local write "Avg Counts/s"(w3202) -> ()
                                }
                                frame Enabled {
                                }
                                }
                                }
                                frame #2 {
                                w3210 = u16 0 items=["Stream to disk", "Post process", "real time process"] ("Ring")
                                n883 = local read "T3R Data processing"() -> (w3209:u16)
                                n884 = local read "save\ndata"() -> (w3212:bool)
                                n885 = Equal?(x=w3209, y=w3210) -> (x = y?=w3208:bool)
                                n886 = Not(x=w3208) -> (.not. x?=w3213:bool)
                                n887 = And(x=w3212, y=w3213) -> (x .and. y?=w3211:bool)
                                n888 = case shown="True" w3211 {
                                tunnel: w3214 -> [_ w3216]
                                frame False {
                                }
                                frame True {
                                n889 = local read "filename prefix"() -> (w3217:string)
                                n890 = local read "data dir"() -> (w3222:path)
                                n891 = call "2pparameters.vi"("command"="get") -> ("params out"=w3237:T10)  [unwired: 1 in]
                                n892 = call "generatedatafilename.vi"("timestamp"=w3216, "filename prefix in"=w3217) -> ("full-filename"=w3215:string)
                                n893 = Unbundle By Name(w3237) -> ("srate"=w3235:sgl, "sAOxy"=w3234:i32, "Xpixels Img"=w3232:i32, "Ypixels Img"=w3230:i32)
                                n894 = Concatenate Strings(w3215, ".lvpt3img" ("string")) -> (w3220:string)
                                n895 = Build Path(base path=w3222, name or relative path=w3220) -> (appended path=w3219:path)
                                n896 = To Unsigned Long Integer(number=w3235) -> (unsigned 32bit integer=w3236:u32)
                                n897 = To Unsigned Long Integer(number=w3234) -> (unsigned 32bit integer=w3233:u32)
                                n898 = To Unsigned Long Integer(number=w3232) -> (unsigned 32bit integer=w3231:u32)
                                n899 = To Unsigned Long Integer(number=w3230) -> (unsigned 32bit integer=w3229:u32)
                                n900 = call "PH-temp-raw.vi"("command"="get") -> ("array out"=w3228:u32[])  [unwired: 1 in]
                                n901 = Build Array (concatenate)(w3236, w3233, w3231, w3229, w3228) -> (w3227:u32[])
                                n902 = Open/Create/Replace File(file path (use dialog)=w3219, operation (0:open)=T8."replace or create") -> (refnum out=w3226:refnum<file>, error out=w3225:errorcluster)  [unwired: 4 in, 1 out]
                                n903 = Write to Binary File(file (use dialog)=w3226, data=w3227, error in=w3225, 5:FALSE ("prepend array or string size? (T)")) -> (refnum out=w3223:refnum<file>, error out=w3224:errorcluster)  [unwired: 2 in, 1 out]
                                n904 = Close File(refnum=w3223, error in=w3224) -> ()  [unwired: 2 out]
                                }
                                }
                                n905 = call "stoperaseLT_img.vi"() -> ()  [unwired: 1 in]
                                }
                                frame #3 {
                                w3243 = u16 1 items=["Stream to disk", "Post process", "real time process"] ("Ring")
                                n906 = local read "T3R Data processing"() -> (w3242:u16)
                                n907 = Equal?(x=w3242, y=w3243) -> (x = y?=w3241:bool)
                                n908 = case shown="True" w3241 {
                                frame False {
                                }
                                frame True {
                                # "intensity"
                                # "lifetime"
                                # "intensity"
                                n909 = property on="img_CH1" class="IntGraph (strict)"() -> ("Value"=w3256:sgl[][])  [unwired: 2 in, 2 out]
                                n910 = Array Max & Min(array=w3256) -> (max value=w3257:sgl)  [unwired: 3 out]
                                n911 = local read "lineshift"() -> (w3244:i32)
                                n912 = local read "min phot"() -> (w3258:u32)
                                n913 = To Unsigned Long Integer(number=w3257) -> (unsigned 32bit integer=w3260:u32)
                                n914 = local read "counts"() -> (w3246:i32)
                                n915 = call "wrapcutlifetime.vi"("lineshift"=w3244) -> ("pt3img"=w3255:u16[][], "lifetimes"=w3253:sgl[][], "okay"=w3248:bool, "# of frames"=w3245:i32)
